vi "CSTK_MCListbox_Designer_Dialog.vi"(10 "MCListbox引用句柄":refnum<vi>, 11 "VI引用输入":refnum<vi>) -> (3 "VI引用输出":refnum<vi>)   [LabVIEW 2015, in "CSTK_MCListbox Designer.lvlib"]
uses:
  CSTK_MCListbox Designer.lvlib
  _CSTK_MCListbox_Designer_ColHdr.ctl
  _CSTK_MCListbox_Designer_ColHdr_Selected.ctl
  _CSTK_MCListbox_Designer_RowAttr.ctl
  <vilib>/Utility/miscctls.llb/LVRowAndColumnTypeDef.ctl
  user32.dll
panel:
  in  "Shutdown":bool
  in  "Minimize":bool
  in  "更新其他属性":bool
  in  "更新表头属性列表":bool
  in  "Refresh":bool
  in  "ArrowDown":bool
  in  "ArrowUp":bool
  in  "Delete":bool
  in  "Create":bool
  in  "行首属性":T1={"宽度"=50, "粗体"=TRUE, "斜体"=FALSE, "对齐"=enum."Center"}
  in  "列":u32
  in  "行":u32
  in  "宽度":u32
  in  "高度":u32
  in  "显示符号":bool
  in  "显示水平线":bool
  in  "显示垂直线":bool
  in  "显示行首":bool
  in  "显示列首":bool
  in  "显示水平滚动条":bool
  in  "显示垂直滚动条":bool
  in  "表头统一属性":T2={"列名称"="", "单元格宽度"=50, "粗体"=TRUE, "斜体"=FALSE, "对齐"=enum."Center"}
  in  "表头属性列表":T3[](array[typedef])
  out "标签名称":string
  # "MCListbox Designer"
  # "列名"
  # "列宽"
  # "粗"
  # "斜"
  # "对齐"
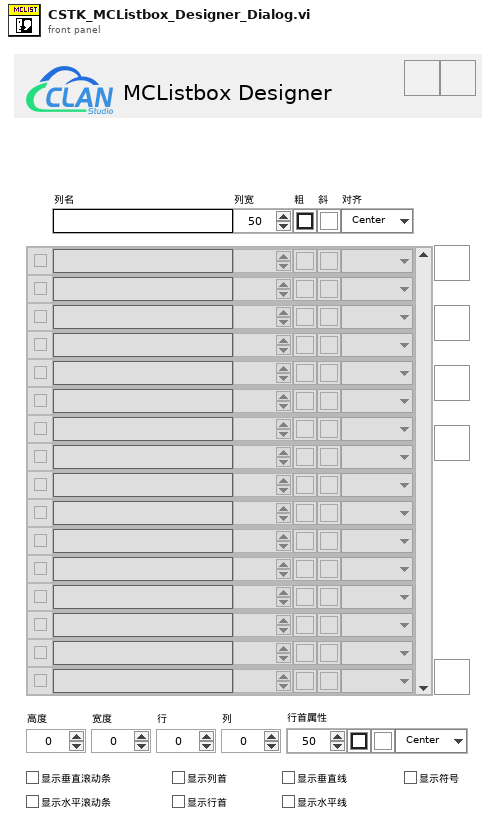
[diagram p1: front panel]
types:
  T1 = typedef "CSTK_MCListbox Designer.lvlib/_CSTK_MCListbox_Designer_RowAttr.ctl" = cluster{"宽度":u32, "粗体":bool, "斜体":bool, "对齐":enum16{"Left", "Center", "Right"}}
  T2 = typedef "CSTK_MCListbox Designer.lvlib/_CSTK_MCListbox_Designer_ColHdr.ctl" = cluster{"列名称":string, "单元格宽度":u32, "粗体":bool, "斜体":bool, "对齐":enum16{"Left", "Center", "Right"}}
  T3 = typedef "CSTK_MCListbox Designer.lvlib/_CSTK_MCListbox_Designer_ColHdr_Selected.ctl" = cluster{"选择":bool, "表头属性":T2}
  T4 = enum32{"Invalid", "Standard", "Closed", "Hidden", "Minimized", "Maximized"}
  T5 = typedef "LVRowAndColumnTypeDef.ctl" = cluster{"Row":i32, "Column":i32}
  T6 = cluster{"高度":refnum<vi>, "宽度":refnum<vi>, "行":refnum<vi>, "列":refnum<vi>, "显示垂直滚动条":refnum<vi>, "显示水平滚动条":refnum<vi>, "显示列首":refnum<vi>, "显示行首":refnum<vi>, "显示垂直线":refnum<vi>, "显示水平线":refnum<vi>, "显示符号":refnum<vi>, "行首属性":refnum<vi>}
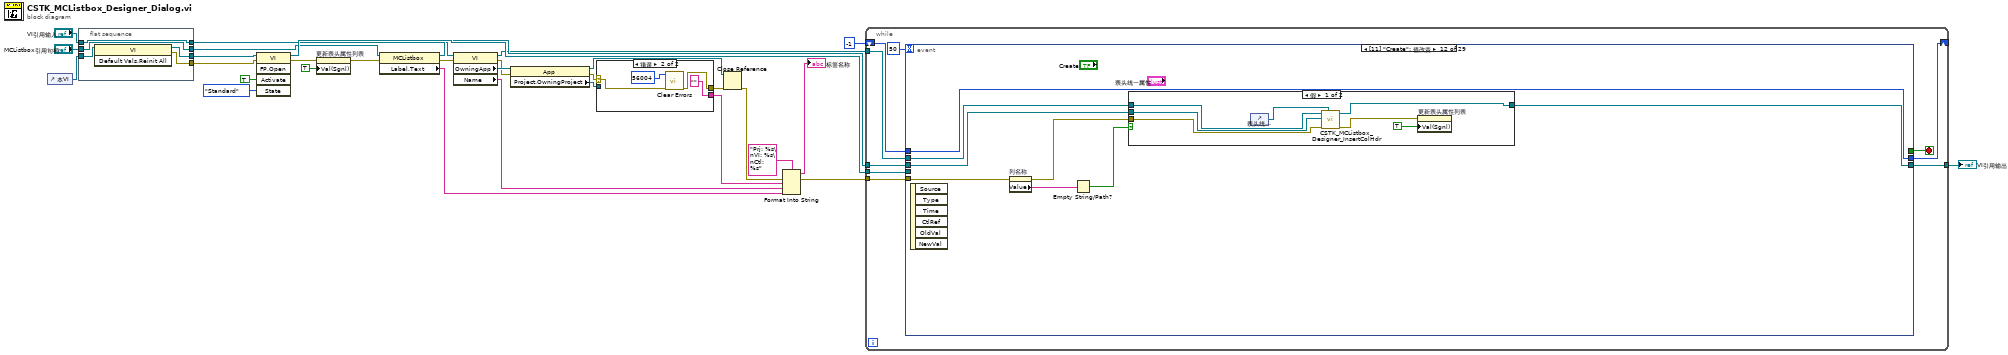
[diagram p0: block diagram]
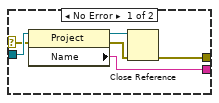
[diagram p2: hidden frame]
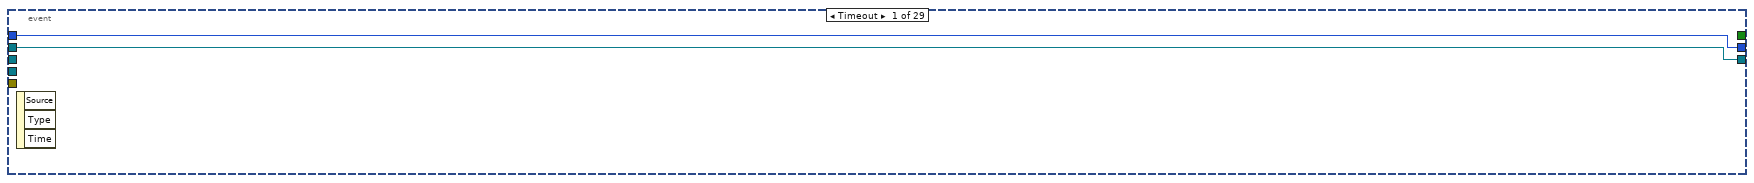
[diagram p3: hidden frame]
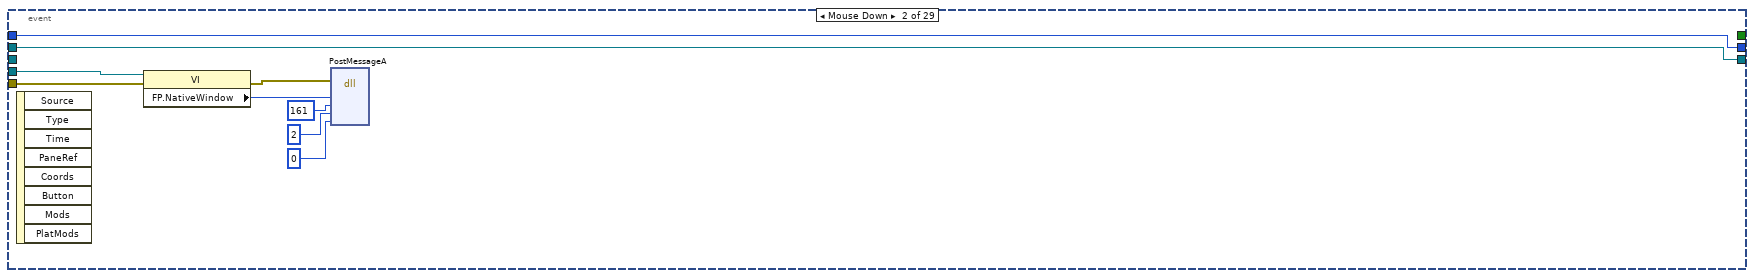
[diagram p4: hidden frame]
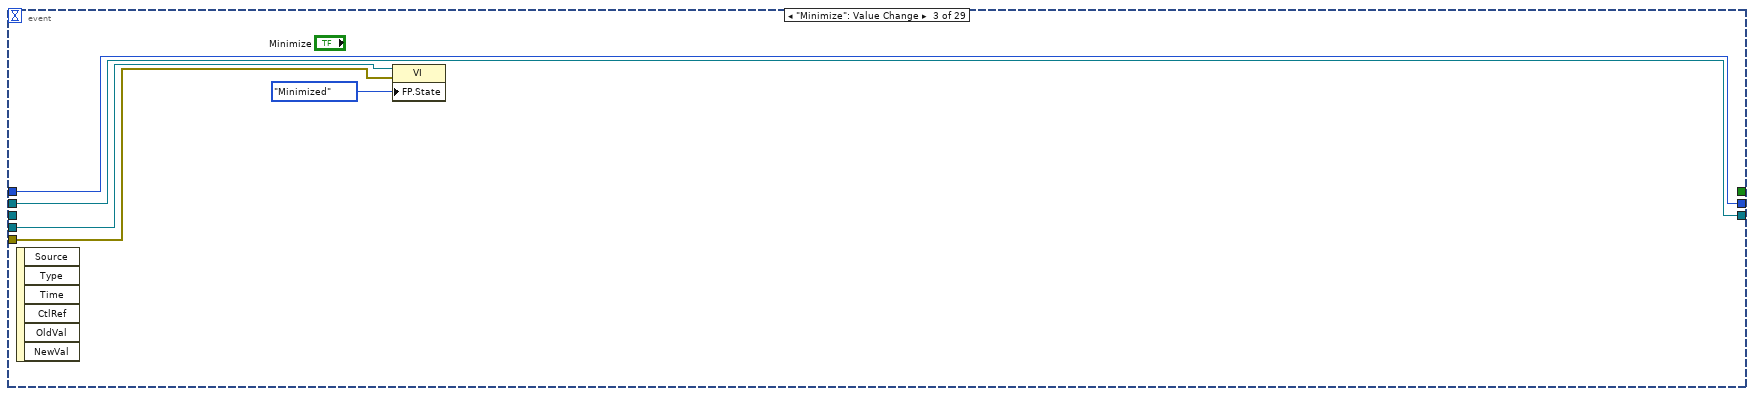
[diagram p5: hidden frame]
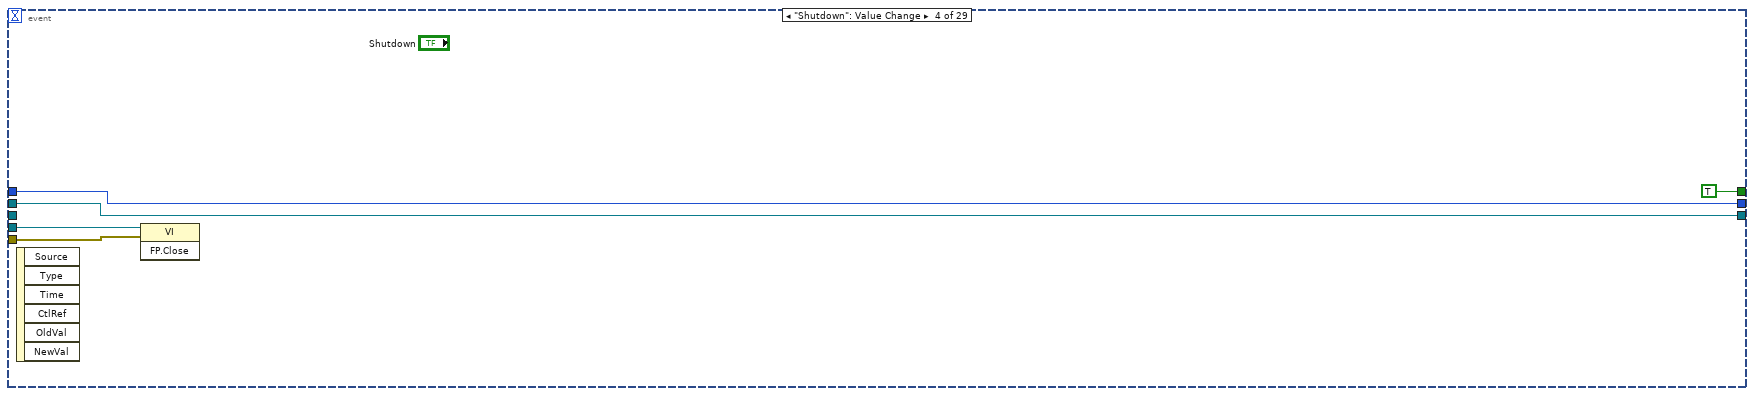
[diagram p6: hidden frame]
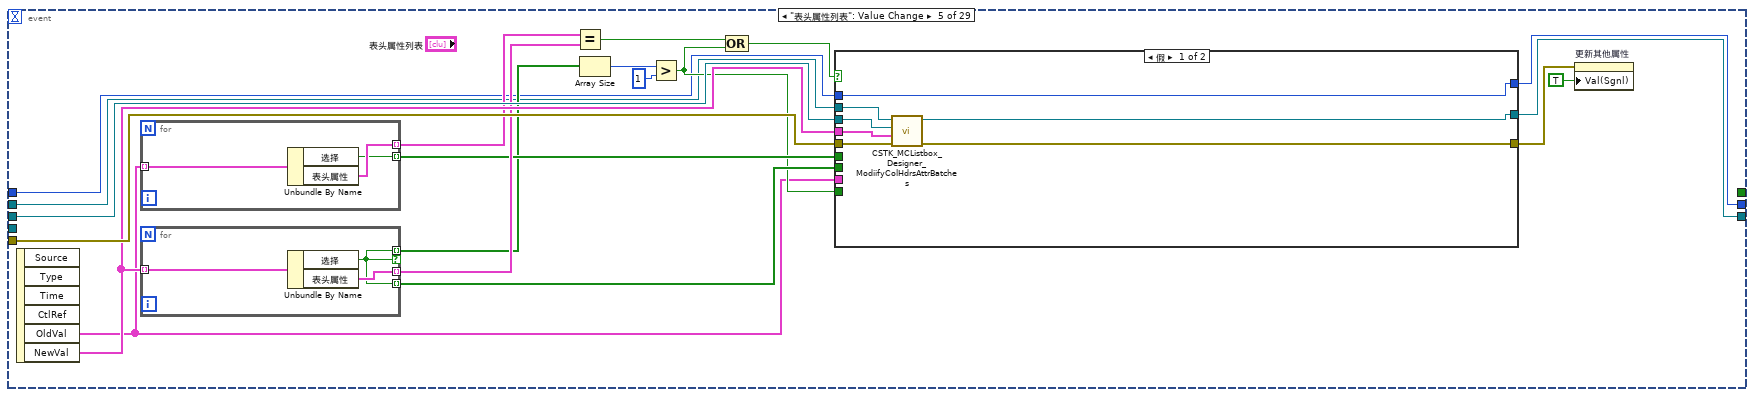
[diagram p7: hidden frame]
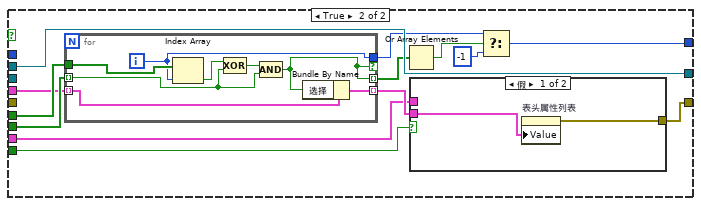
[diagram p8: hidden frame]
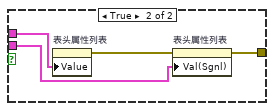
[diagram p9: hidden frame]
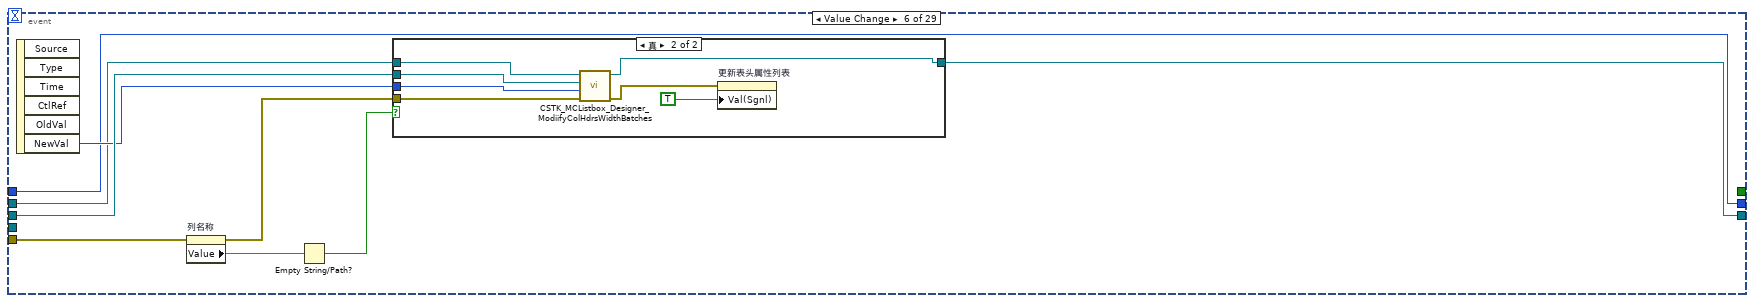
[diagram p10: hidden frame]
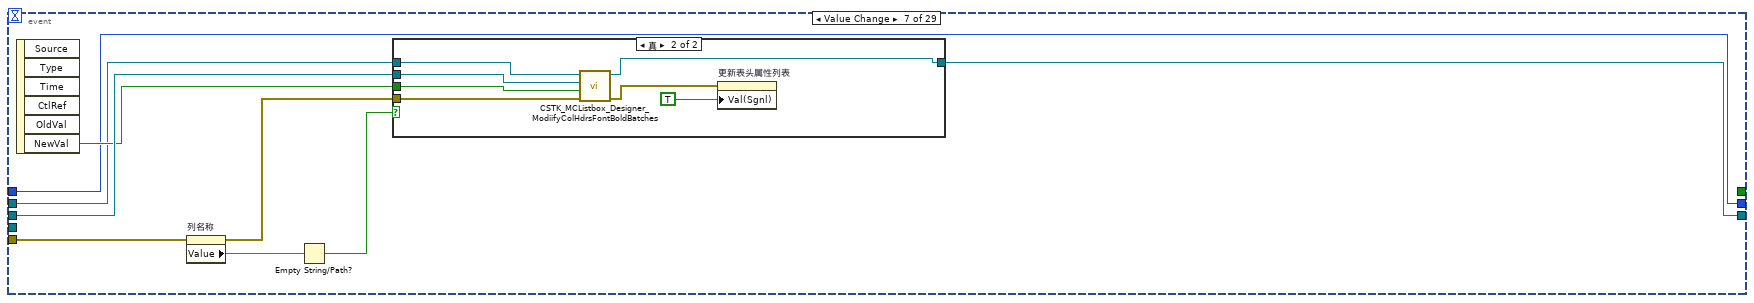
[diagram p12: hidden frame]
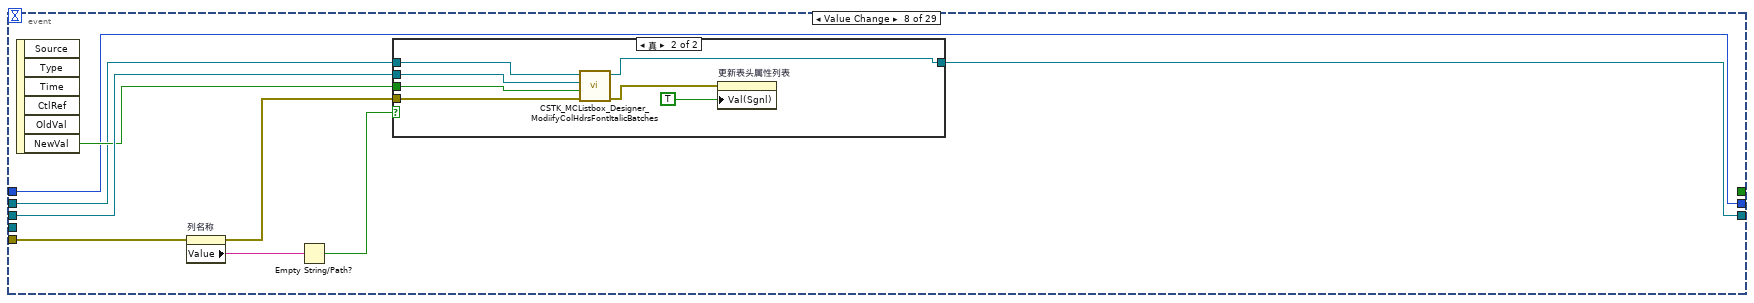
[diagram p14: hidden frame]
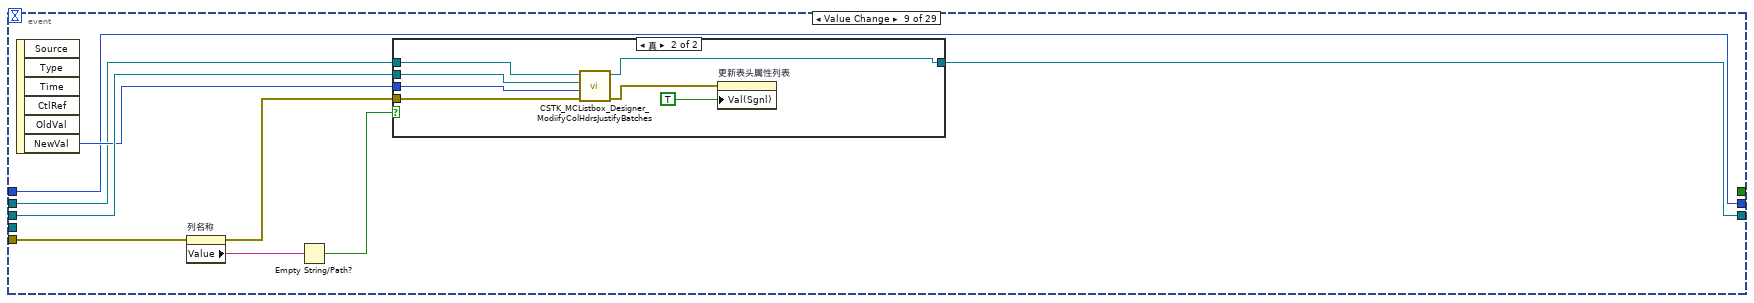
[diagram p16: hidden frame]
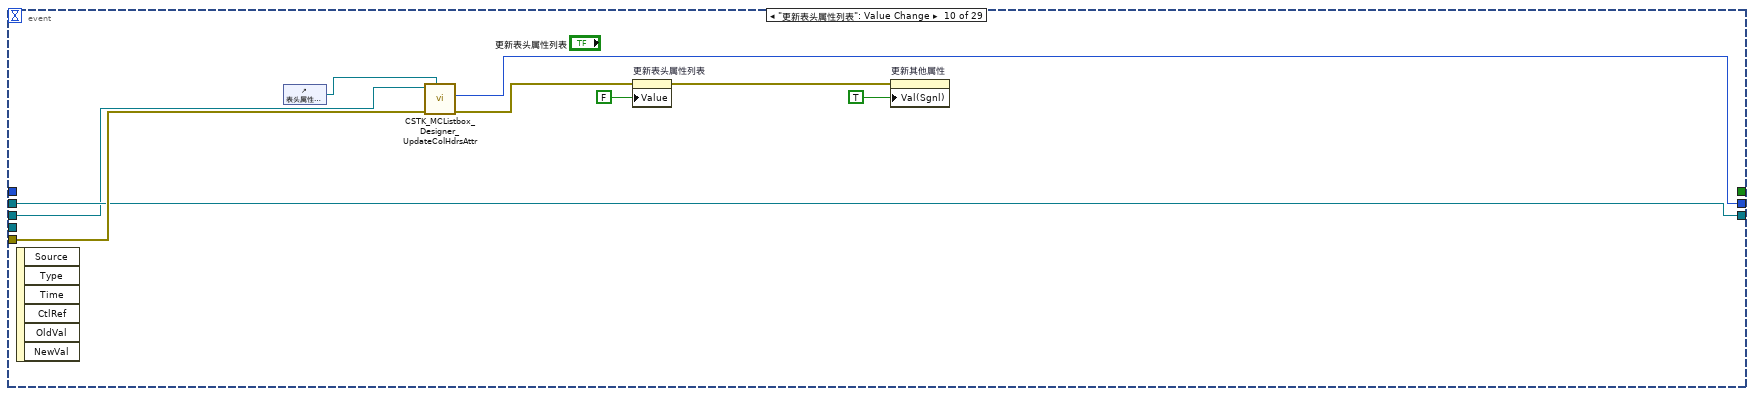
[diagram p18: hidden frame]
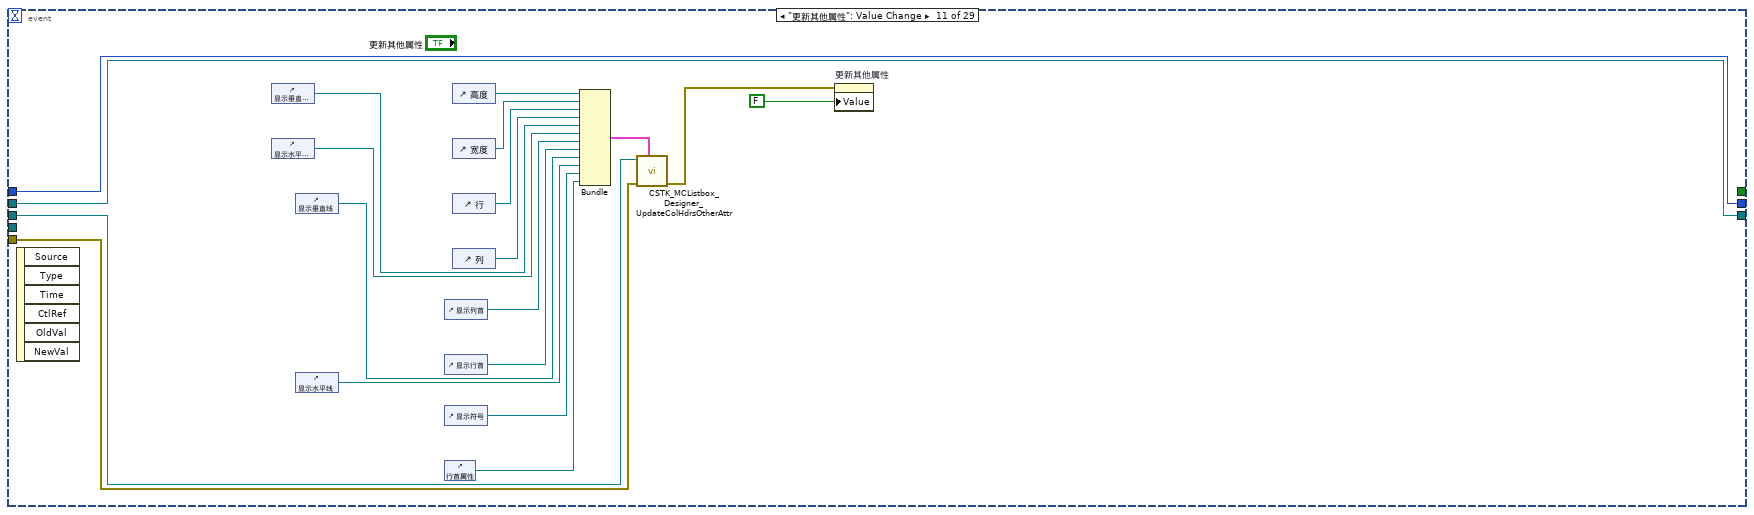
[diagram p19: hidden frame]
diagram:
  n1 = control-ref of="本VI"() -> (w31:refnum<vi>)
  n2 = flat-sequence {
    tunnel: w31 -> [w36]
    tunnel: [w35] -> w30
    tunnel: [w34] -> w29
    tunnel: [w32] -> w19
    tunnel: "MCListbox引用句柄" -> [w32]
    tunnel: [w33] -> w6
    tunnel: "VI引用输入" -> [w33]
    frame #0 {
      n3 = invoke class="VI" method="Default Vals.Reinit All"(reference=w36) -> (reference out=w34:refnum<vi>, error out=w35:errorcluster)  [unwired: 2 in, 1 out]
    }
  }
  n4 = invoke class="VI" method="FP.Open"(reference=w29, error in=w30, "Activate"=TRUE ("激活？"), "State"=T4."Standard" ("状态")) -> (reference out=w20:refnum<vi>, error out=w21:errorcluster)  [unwired: 1 in, 3 out]
  n5 = property on="更新表头属性列表" class="Bool (严格)"(error in=w21, "Val(Sgnl)"=TRUE ("值(信号)")) -> (error out=w1:errorcluster)  [unwired: 1 in, 1 out]
  n6 = property class="MCListbox"(reference=w19, error in=w1) -> (reference out=w18:refnum<vi>, error out=w9:errorcluster, "Label.Text"=w12:string)
  n7 = property class="VI"(reference=w6, error in=w9) -> (reference out=w14:refnum<vi>, error out=w11:errorcluster, "OwningApp"=w17:refnum<vi>, "Name"=w15:string)
  n8 = property class="App"(reference=w17, error in=w11) -> (reference out=w10:refnum<vi>, error out=w4:errorcluster, "Project.OwningProject"=w5:refnum<vi>)
  n9 = case shown="错误" w4 {
    selector: w4 -> [w41 w45]
    tunnel: w5 -> [w42 _]
    tunnel: [w38 "" ("Name")] -> w3
    tunnel: [w37 w44] -> w2
    frame No Error {
      n10 = property class="Project"(reference=w42, error in=w41) -> (reference out=w39:refnum<vi>, error out=w40:errorcluster, "Name"=w38:string)
      n11 = Close Reference(reference=w39, error in (no error)=w40) -> (error out=w37:errorcluster)
    }
    frame Error {
      n12 = call <vilib>:"Clear Errors.vi"("error in (no error)"=w45, "specific error code to clear (0: all)"=56004) -> ("error out"=w44:errorcluster)  [unwired: 4 in, 1 out]
    }
  }
  n13 = Close Reference(reference=w10, error in (no error)=w2) -> (error out=w8:errorcluster)
  n14 = Format Into String(format string="Prj: %s\nVI: %s\nCtl: %s" ("格式字符串"), error in=w8, w3, w15, w12) -> (resulting string=→"标签名称":string, error out=w7:errorcluster)  [unwired: 1 in]
  n15 = while {
    tunnel: w18 -> [w53]
    tunnel: w7 -> [w52]
    tunnel: w14 -> [w50]
    tunnel: [w51] -> w25
    shift-right: [w49] -> _
    shift-left: -1 -> [w48]
    tunnel: w20 -> [w47]
    stop <- w55 stop-if-true
    n16 = event shown="[11] \"Create\": 值改变" {
      selector: _ -> [_ _ _ _ _ _ _ _ _ _ _ _ _ _ _ _ _ _ _ _ _ _ _ _ _ _ _ _ _]
      dyn-events: _ -> [_ _ _ _ _ _ _ _ _ _ _ _ _ _ _ _ _ _ _ _ _ _ _ _ _ _ _ _ _]
      timeout: 50 -> [_ _ _ _ _ _ _ _ _ _ _ _ _ _ _ _ _ _ _ _ _ _ _ _ _ _ _ _ _]
      tunnel: [_ _ _ TRUE _ _ _ _ _ _ _ _ _ _ _ _ _ _ _ _ _ _ _ _ _ _ _ _ TRUE] -> w55
      tunnel: w53 -> [_ _ _ _ w96 w145 w162 w179 w196 w208 w228 w240 w251 w266 w281 _ w302 w309 w316 w323 w330 w337 w344 w351 w358 w365 w372 w383 _]
      tunnel: w52 -> [_ w58 w68 w73 w95 w144 w161 w178 w195 w211 w230 w239 w250 w265 w280 w294 w301 w308 w315 w322 w329 w336 w343 w350 w357 w364 w371 w382 _]
      tunnel: [w57 w66 w71 w76 w79 w138 w155 w172 w189 w210 w229 w235 w252 w267 w282 w297 w304 w311 w318 w325 w332 w339 w346 w353 w360 w367 w374 w386 w388] -> w51
      tunnel: w50 -> [w57 w66 w71 w76 w80 w139 w156 w173 w190 w210 w229 w236 w253 w268 w283 w297 w304 w311 w318 w325 w332 w339 w346 w353 w360 w367 w374 w386 w388]
      tunnel: [w56 w65 w70 w75 w81 w137 w154 w171 w188 w209 w227 w233 w249 w264 w279 w296 w303 w310 w317 w324 w331 w338 w345 w352 w359 w366 w373 w385 w387] -> w49
      tunnel: w48 -> [w56 w65 w70 w75 w82 w137 w154 w171 w188 _ w227 w233 w249 w264 w279 w296 w303 w310 w317 w324 w331 w338 w345 w352 w359 w366 w373 w385 w387]
      tunnel: w47 -> [_ w59 w67 w74 _ _ _ _ _ _ _ _ _ _ _ _ _ _ _ _ _ _ _ _ _ _ _ _ _]
      event Timeout {
        n17 = event-data() -> ()  [unwired: 1 in, 3 out]
      }
      event Mouse Down {
        n18 = event-data() -> ()  [unwired: 1 in, 8 out]
        n19 = property class="VI"(reference=w59, error in=w58) -> (error out=w60:errorcluster, "FP.NativeWindow"=w61:u64)  [unwired: 1 out]
        n20 = dll-call lib="user32.dll" fn="PostMessageA"(error in=w60, "hWnd"=w61, "Msg"=161, "wParam"=2, "IParam"=0 ("wParam")) -> ()  [unwired: 7 in, 2 out]
      }
      event "Minimize": Value Change {
        n21 = event-data() -> ()  [unwired: 1 in, 6 out]
        n22 = property class="VI"(reference=w67, error in=w68, "FP.State"=T4."Minimized" ("Front Panel Window:State")) -> ()  [unwired: 2 out]
      }
      event "Shutdown": Value Change {
        n23 = event-data() -> ()  [unwired: 1 in, 6 out]
        n24 = invoke class="VI" method="FP.Close"(reference=w74, error in=w73) -> ()  [unwired: 1 in, 3 out]
      }
      event "表头属性列表": Value Change {
        n25 = event-data() -> ("OldVal"=w83:T3[], "NewVal"=w94:T3[])  [unwired: 1 in, 4 out]
        n26 = for {
          tunnel: w83 -> [w102] mode=indexing
          tunnel: [w101] -> w93 mode=indexing
          tunnel: [w100] -> w90 mode=indexing
          n27 = Unbundle By Name(w102) -> ("选择"=w100:bool, "表头属性"=w101:T2)
        }
        n28 = for {
          tunnel: w94 -> [w99] mode=indexing
          tunnel: [w98] -> w92 mode=indexing
          tunnel: [w97] -> w89 mode=indexing
          tunnel: [w97] -> w88 mode=indexing if=w97
          n29 = Unbundle By Name(w99) -> ("选择"=w97:bool, "表头属性"=w98:T2)
        }
        n30 = Equal?(x=w93, y=w92) -> (x = y?=w91:bool)
        n31 = Array Size(array=w88) -> (size(s)=w86:i32)
        n32 = Greater?(x=w86, y=1) -> (0:w84:bool)
        n33 = Compound Arithmetic op=OR ("复合运算")(w91, w84) -> (w87:bool)
        n34 = case shown="假" w87 {
          tunnel: w96 -> [w104 _]
          tunnel: w94 -> [w109 w120]
          tunnel: w80 -> [w105 w116]
          tunnel: w95 -> [w108 _]
          tunnel: w90 -> [_ w122]
          tunnel: w89 -> [_ w121]
          tunnel: w84 -> [_ w118]
          tunnel: w83 -> [_ w117]
          tunnel: w82 -> [w107 _]
          tunnel: [w107 w112] -> w81
          tunnel: [w106 w116] -> w79
          tunnel: [w103 w110] -> w77
          frame False {
            n35 = call "CSTK_MCListbox_Designer_ModiifyColHdrsAttrBatches.vi"("错误输入（无错误）"=w108, "Attr"=w109, "MulticolumnListbox输入"=w104, "VI输入"=w105) -> ("错误输出"=w103:errorcluster, "VI输出"=w106:refnum<vi>)  [unwired: 6 in]
          }
          frame True {
            n36 = for {
              tunnel: w122 -> [w135]
              tunnel: w121 -> [w134] mode=indexing
              tunnel: w120 -> [w132] mode=indexing
              tunnel: [w131] -> w119 mode=indexing
              tunnel: [w130] -> w113 if=w129
              tunnel: [w129] -> w115 mode=indexing
              i -> [w130]
              n37 = Index Array(array=w135, index=w130) -> (element=w133:bool)
              n38 = Compound Arithmetic op=XOR ("复合运算")(w133, w134) -> (w136:bool)
              n39 = Compound Arithmetic op=AND ("复合运算")(w136, w134) -> (w129:bool)
              n40 = Bundle By Name(cluster=w132, "选择"=w129) -> (w131:T3)
            }
            n41 = Or Array Elements(Boolean array=w115) -> (logical OR=w114:bool)
            n42 = case shown="假" w118 {
              tunnel: w119 -> [w124 w127]
              tunnel: w117 -> [_ w126]
              tunnel: [w123 w125] -> w110
              frame False {
                n43 = property on="表头属性列表" class="Arr (严格)"("Value"=w124) -> (error out=w123:errorcluster)  [unwired: 2 in, 1 out]
              }
              frame True {
                n44 = property on="表头属性列表" class="Arr (严格)"("Value"=w126) -> (error out=w128:errorcluster)  [unwired: 2 in, 1 out]
                n45 = property on="表头属性列表" class="Arr (严格)"(error in=w128, "Val(Sgnl)"=w127) -> (error out=w125:errorcluster)  [unwired: 1 in, 1 out]
              }
            }
            n46 = Select(t=w113, s=w114, f=-1) -> (s? t:f=w112:i32)
          }
        }
        n47 = property on="更新其他属性" class="Bool (严格)"(error in=w77, "Val(Sgnl)"=TRUE ("值(信号)")) -> ()  [unwired: 1 in, 2 out]
      }
      event Value Change {
        n48 = event-data() -> ("NewVal"=w140:u32)  [unwired: 1 in, 5 out]
        n49 = property on="列名称" class="Str"(error in=w144) -> (error out=w143:errorcluster, "Value"=w142:string)  [unwired: 1 in, 1 out]
        n50 = Empty String/Path?(string/path=w142) -> (empty?=w141:bool)
        n51 = case shown="真" w141 {
          tunnel: w145 -> [_ w147]
          tunnel: w143 -> [_ w152]
          tunnel: w140 -> [_ w153]
          tunnel: w139 -> [w146 w148]
          tunnel: [w146 w151] -> w138
          frame False {
          }
          frame True {
            n52 = call "CSTK_MCListbox_Designer_ModiifyColHdrsWidthBatches.vi"("错误输入（无错误）"=w152, "Width"=w153, "MulticolumnListbox输入"=w147, "VI输入"=w148) -> ("错误输出"=w149:errorcluster, "VI输出"=w151:refnum<vi>)  [unwired: 6 in]
            n53 = property on="更新表头属性列表" class="Bool (严格)"(error in=w149, "Val(Sgnl)"=TRUE ("值(信号)")) -> ()  [unwired: 1 in, 2 out]
          }
        }
      }
      event Value Change {
        n54 = event-data() -> ("NewVal"=w157:bool)  [unwired: 1 in, 5 out]
        n55 = property on="列名称" class="Str"(error in=w161) -> (error out=w160:errorcluster, "Value"=w159:string)  [unwired: 1 in, 1 out]
        n56 = Empty String/Path?(string/path=w159) -> (empty?=w158:bool)
        n57 = case shown="真" w158 {
          tunnel: w162 -> [_ w164]
          tunnel: w160 -> [_ w169]
          tunnel: w157 -> [_ w170]
          tunnel: w156 -> [w163 w165]
          tunnel: [w163 w168] -> w155
          frame False {
          }
          frame True {
            n58 = call "CSTK_MCListbox_Designer_ModiifyColHdrsFontBoldBatches.vi"("错误输入（无错误）"=w169, "FontBold"=w170, "MulticolumnListbox输入"=w164, "VI输入"=w165) -> ("错误输出"=w166:errorcluster, "VI输出"=w168:refnum<vi>)  [unwired: 6 in]
            n59 = property on="更新表头属性列表" class="Bool (严格)"(error in=w166, "Val(Sgnl)"=TRUE ("值(信号)")) -> ()  [unwired: 1 in, 2 out]
          }
        }
      }
      event Value Change {
        n60 = event-data() -> ("NewVal"=w174:bool)  [unwired: 1 in, 5 out]
        n61 = property on="列名称" class="Str"(error in=w178) -> (error out=w177:errorcluster, "Value"=w176:string)  [unwired: 1 in, 1 out]
        n62 = Empty String/Path?(string/path=w176) -> (empty?=w175:bool)
        n63 = case shown="真" w175 {
          tunnel: w179 -> [_ w181]
          tunnel: w177 -> [_ w186]
          tunnel: w174 -> [_ w187]
          tunnel: w173 -> [w180 w182]
          tunnel: [w180 w185] -> w172
          frame False {
          }
          frame True {
            n64 = call "CSTK_MCListbox_Designer_ModiifyColHdrsFontItalicBatches.vi"("错误输入（无错误）"=w186, "FontItalic"=w187, "MulticolumnListbox输入"=w181, "VI输入"=w182) -> ("错误输出"=w183:errorcluster, "VI输出"=w185:refnum<vi>)  [unwired: 6 in]
            n65 = property on="更新表头属性列表" class="Bool (严格)"(error in=w183, "Val(Sgnl)"=TRUE ("值(信号)")) -> ()  [unwired: 1 in, 2 out]
          }
        }
      }
      event Value Change {
        n66 = event-data() -> ("NewVal"=w191:enum16{"Left", "Center", "Right"})  [unwired: 1 in, 5 out]
        n67 = property on="列名称" class="Str"(error in=w195) -> (error out=w194:errorcluster, "Value"=w193:string)  [unwired: 1 in, 1 out]
        n68 = Empty String/Path?(string/path=w193) -> (empty?=w192:bool)
        n69 = case shown="真" w192 {
          tunnel: w196 -> [_ w199]
          tunnel: w194 -> [_ w203]
          tunnel: w191 -> [_ w204]
          tunnel: w190 -> [w197 w198]
          tunnel: [w197 w202] -> w189
          frame False {
          }
          frame True {
            n70 = call "CSTK_MCListbox_Designer_ModiifyColHdrsJustifyBatches.vi"("错误输入（无错误）"=w203, "Justify"=w204, "MulticolumnListbox输入"=w199, "VI输入"=w198) -> ("错误输出"=w200:errorcluster, "VI输出"=w202:refnum<vi>)  [unwired: 6 in]
            n71 = property on="更新表头属性列表" class="Bool (严格)"(error in=w200, "Val(Sgnl)"=TRUE ("值(信号)")) -> ()  [unwired: 1 in, 2 out]
          }
        }
      }
      event "更新表头属性列表": Value Change {
        n72 = event-data() -> ()  [unwired: 1 in, 6 out]
        n73 = control-ref of="表头属性列表"() -> (w205:refnum<vi>)
        n74 = call "CSTK_MCListbox_Designer_UpdateColHdrsAttr.vi"("表头属性列表输入"=w205, "错误输入（无错误）"=w211, "MCListbox引用句柄"=w208) -> ("错误输出"=w213:errorcluster, "Selected Index"=w209:i32)  [unwired: 7 in]
        n75 = property on="更新表头属性列表" class="Bool (严格)"(error in=w213, "Value"=FALSE ("更新表头属性列表")) -> (error out=w207:errorcluster)  [unwired: 1 in, 1 out]
        n76 = property on="更新其他属性" class="Bool (严格)"(error in=w207, "Val(Sgnl)"=TRUE ("值(信号)")) -> ()  [unwired: 1 in, 2 out]
      }
      event "更新其他属性": Value Change {
        n77 = event-data() -> ()  [unwired: 1 in, 6 out]
        n78 = control-ref of="显示垂直滚动条"() -> (w220:refnum<vi>)
        n79 = control-ref of="显示水平滚动条"() -> (w221:refnum<vi>)
        n80 = control-ref of="显示垂直线"() -> (w224:refnum<vi>)
        n81 = control-ref of="显示水平线"() -> (w225:refnum<vi>)
        n82 = control-ref of="显示列首"() -> (w222:refnum<vi>)
        n83 = control-ref of="显示行首"() -> (w223:refnum<vi>)
        n84 = control-ref of="显示符号"() -> (w226:refnum<vi>)
        n85 = control-ref of="行首属性"() -> (w214:refnum<vi>)
        n86 = control-ref of="高度"() -> (w216:refnum<vi>)
        n87 = control-ref of="宽度"() -> (w217:refnum<vi>)
        n88 = control-ref of="行"() -> (w218:refnum<vi>)
        n89 = control-ref of="列"() -> (w219:refnum<vi>)
        n90 = Bundle("高度"=w216, "宽度"=w217, "行"=w218, "列"=w219, "显示垂直滚动条"=w220, "显示水平滚动条"=w221, "显示列首"=w222, "显示行首"=w223, "显示垂直线"=w224, "显示水平线"=w225, "显示符号"=w226, "行首属性"=w214) -> (w215:T6)  [unwired: 1 in]
        n91 = call "CSTK_MCListbox_Designer_UpdateColHdrsOtherAttr.vi"("引用输入"=w215, "错误输入（无错误）"=w230, "MCListbox引用句柄"=w228) -> ("错误输出"=w232:errorcluster)  [unwired: 8 in]
        n92 = property on="更新其他属性" class="Bool (严格)"(error in=w232, "Value"=FALSE ("更新表头属性列表")) -> ()  [unwired: 1 in, 2 out]
      }
      event "Create": Value Change {
        n93 = event-data() -> ()  [unwired: 1 in, 6 out]
        n94 = property on="列名称" class="Str"(error in=w239) -> (error out=w238:errorcluster, "Value"=w234:string)  [unwired: 1 in, 1 out]
        n95 = Empty String/Path?(string/path=w234) -> (empty?=w237:bool)
        n96 = case shown="假" w237 {
          tunnel: w240 -> [w245 _]
          tunnel: w238 -> [w247 _]
          tunnel: w236 -> [w242 w248]
          tunnel: [w246 w248] -> w235
          frame False {
            n97 = control-ref of="表头统一属性"() -> (w241:refnum<vi>)
            n98 = call "CSTK_MCListbox_Designer_InsertColHdr.vi"("表头统一属性输入"=w241, "错误输入（无错误）"=w247, "MCListbox引用句柄"=w245, "VI输入"=w242) -> ("错误输出"=w243:errorcluster, "VI输出"=w246:refnum<vi>)  [unwired: 6 in]
            n99 = property on="更新表头属性列表" class="Bool (严格)"(error in=w243, "Val(Sgnl)"=TRUE ("值(信号)")) -> ()  [unwired: 1 in, 2 out]
          }
          frame True {
          }
        }
      }
      event "Delete": Value Change {
        n100 = event-data() -> ()  [unwired: 1 in, 6 out]
        n101 = Greater Or Equal To 0?(x=w249) -> (x >= 0?=w254:bool)
        n102 = case shown="真" w254 {
          tunnel: w251 -> [_ w259]
          tunnel: w250 -> [_ w263]
          tunnel: w253 -> [w255 w257]
          tunnel: [w255 w262] -> w252
          tunnel: w249 -> [_ w256]
          frame False {
          }
          frame True {
            n103 = control-ref of="表头属性列表"() -> (w258:refnum<vi>)
            n104 = call "CSTK_MCListbox_Designer_DeleteColHdr.vi"("表头属性列表输入"=w258, "错误输入（无错误）"=w263, "Selected Index"=w256, "MCListbox引用句柄"=w259, "VI输入"=w257) -> ("错误输出"=w260:errorcluster, "VI输出"=w262:refnum<vi>)  [unwired: 5 in]
            n105 = property on="更新表头属性列表" class="Bool (严格)"(error in=w260, "Val(Sgnl)"=TRUE ("值(信号)")) -> ()  [unwired: 1 in, 2 out]
          }
        }
      }
      event "ArrowUp": Value Change {
        n106 = event-data() -> ()  [unwired: 1 in, 6 out]
        n107 = Greater Or Equal To 0?(x=w264) -> (x >= 0?=w269:bool)
        n108 = case shown="真" w269 {
          tunnel: w266 -> [_ w274]
          tunnel: w265 -> [_ w278]
          tunnel: w268 -> [w270 w272]
          tunnel: [w270 w277] -> w267
          tunnel: w264 -> [_ w271]
          frame False {
          }
          frame True {
            n109 = control-ref of="表头属性列表"() -> (w273:refnum<vi>)
            n110 = call "CSTK_MCListbox_Designer_MoveUpColHdr.vi"("表头属性列表输入"=w273, "错误输入（无错误）"=w278, "Selected Index"=w271, "MCListbox引用句柄"=w274, "VI输入"=w272) -> ("错误输出"=w275:errorcluster, "VI输出"=w277:refnum<vi>)  [unwired: 5 in]
            n111 = property on="更新表头属性列表" class="Bool (严格)"(error in=w275, "Val(Sgnl)"=TRUE ("值(信号)")) -> ()  [unwired: 1 in, 2 out]
          }
        }
      }
      event "ArrowDown": Value Change {
        n112 = event-data() -> ()  [unwired: 1 in, 6 out]
        n113 = Greater Or Equal To 0?(x=w279) -> (x >= 0?=w284:bool)
        n114 = case shown="真" w284 {
          tunnel: w281 -> [_ w289]
          tunnel: w280 -> [_ w293]
          tunnel: w283 -> [w285 w287]
          tunnel: [w285 w292] -> w282
          tunnel: w279 -> [_ w286]
          frame False {
          }
          frame True {
            n115 = control-ref of="表头属性列表"() -> (w288:refnum<vi>)
            n116 = call "CSTK_MCListbox_Designer_MoveDownColHdr.vi"("表头属性列表输入"=w288, "错误输入（无错误）"=w293, "Selected Index"=w286, "MCListbox引用句柄"=w289, "VI输入"=w287) -> ("错误输出"=w290:errorcluster, "VI输出"=w292:refnum<vi>)  [unwired: 5 in]
            n117 = property on="更新表头属性列表" class="Bool (严格)"(error in=w290, "Val(Sgnl)"=TRUE ("值(信号)")) -> ()  [unwired: 1 in, 2 out]
          }
        }
      }
      event "Refresh": Value Change {
        n118 = event-data() -> ()  [unwired: 1 in, 6 out]
        n119 = property on="更新表头属性列表" class="Bool (严格)"(error in=w294, "Val(Sgnl)"=TRUE ("值(信号)")) -> ()  [unwired: 1 in, 2 out]
      }
      event "高度": Value Change {
        n120 = event-data() -> ("NewVal"=w300:u32)  [unwired: 1 in, 5 out]
        n121 = property class="MCListbox"(reference=w302, error in=w301, "Height"=w300) -> (error out=w298:errorcluster)  [unwired: 1 out]
        n122 = property on="更新其他属性" class="Bool (严格)"(error in=w298, "Val(Sgnl)"=TRUE ("值(信号)")) -> ()  [unwired: 1 in, 2 out]
      }
      event "宽度": Value Change {
        n123 = event-data() -> ("NewVal"=w307:u32)  [unwired: 1 in, 5 out]
        n124 = property class="MCListbox"(reference=w309, error in=w308, "Width"=w307) -> (error out=w305:errorcluster)  [unwired: 1 out]
        n125 = property on="更新其他属性" class="Bool (严格)"(error in=w305, "Val(Sgnl)"=TRUE ("值(信号)")) -> ()  [unwired: 1 in, 2 out]
      }
      event "行": Value Change {
        n126 = event-data() -> ("NewVal"=w314:u32)  [unwired: 1 in, 5 out]
        n127 = property class="MCListbox"(reference=w316, error in=w315, "NumRows"=w314) -> (error out=w312:errorcluster)  [unwired: 1 out]
        n128 = property on="更新其他属性" class="Bool (严格)"(error in=w312, "Val(Sgnl)"=TRUE ("值(信号)")) -> ()  [unwired: 1 in, 2 out]
      }
      event "列": Value Change {
        n129 = event-data() -> ("NewVal"=w321:u32)  [unwired: 1 in, 5 out]
        n130 = property class="MCListbox"(reference=w323, error in=w322, "NumCols"=w321) -> (error out=w319:errorcluster)  [unwired: 1 out]
        n131 = property on="更新其他属性" class="Bool (严格)"(error in=w319, "Val(Sgnl)"=TRUE ("值(信号)")) -> ()  [unwired: 1 in, 2 out]
      }
      event "显示垂直滚动条": Value Change {
        n132 = event-data() -> ("NewVal"=w328:bool)  [unwired: 1 in, 5 out]
        n133 = property class="MCListbox"(reference=w330, error in=w329, "VScrollVis"=w328) -> (error out=w326:errorcluster)  [unwired: 1 out]
        n134 = property on="更新其他属性" class="Bool (严格)"(error in=w326, "Val(Sgnl)"=TRUE ("值(信号)")) -> ()  [unwired: 1 in, 2 out]
      }
      event "显示水平滚动条": Value Change {
        n135 = event-data() -> ("NewVal"=w335:bool)  [unwired: 1 in, 5 out]
        n136 = property class="MCListbox"(reference=w337, error in=w336, "HScrollVis"=w335) -> (error out=w333:errorcluster)  [unwired: 1 out]
        n137 = property on="更新其他属性" class="Bool (严格)"(error in=w333, "Val(Sgnl)"=TRUE ("值(信号)")) -> ()  [unwired: 1 in, 2 out]
      }
      event "显示列首": Value Change {
        n138 = event-data() -> ("NewVal"=w342:bool)  [unwired: 1 in, 5 out]
        n139 = property class="MCListbox"(reference=w344, error in=w343, "ColHdrVis"=w342) -> (error out=w340:errorcluster)  [unwired: 1 out]
        n140 = property on="更新其他属性" class="Bool (严格)"(error in=w340, "Val(Sgnl)"=TRUE ("值(信号)")) -> ()  [unwired: 1 in, 2 out]
      }
      event "显示行首": Value Change {
        n141 = event-data() -> ("NewVal"=w349:bool)  [unwired: 1 in, 5 out]
        n142 = property class="MCListbox"(reference=w351, error in=w350, "RowHdrVis"=w349) -> (error out=w347:errorcluster)  [unwired: 1 out]
        n143 = property on="更新其他属性" class="Bool (严格)"(error in=w347, "Val(Sgnl)"=TRUE ("值(信号)")) -> ()  [unwired: 1 in, 2 out]
      }
      event "显示垂直线": Value Change {
        n144 = event-data() -> ("NewVal"=w356:bool)  [unwired: 1 in, 5 out]
        n145 = property class="MCListbox"(reference=w358, error in=w357, "Vertical Lines Visible"=w356) -> (error out=w354:errorcluster)  [unwired: 1 out]
        n146 = property on="更新其他属性" class="Bool (严格)"(error in=w354, "Val(Sgnl)"=TRUE ("值(信号)")) -> ()  [unwired: 1 in, 2 out]
      }
      event "显示水平线": Value Change {
        n147 = event-data() -> ("NewVal"=w363:bool)  [unwired: 1 in, 5 out]
        n148 = property class="MCListbox"(reference=w365, error in=w364, "Horizontal Lines Visible"=w363) -> (error out=w361:errorcluster)  [unwired: 1 out]
        n149 = property on="更新其他属性" class="Bool (严格)"(error in=w361, "Val(Sgnl)"=TRUE ("值(信号)")) -> ()  [unwired: 1 in, 2 out]
      }
      event "显示符号": Value Change {
        n150 = event-data() -> ("NewVal"=w370:bool)  [unwired: 1 in, 5 out]
        n151 = property class="MCListbox"(reference=w372, error in=w371, "Symbols Vis"=w370) -> (error out=w368:errorcluster)  [unwired: 1 out]
        n152 = property on="更新其他属性" class="Bool (严格)"(error in=w368, "Val(Sgnl)"=TRUE ("值(信号)")) -> ()  [unwired: 1 in, 2 out]
      }
      event Value Change {
        n153 = event-data() -> ("NewVal"=w379:T1)  [unwired: 1 in, 5 out]
        n154 = Unbundle By Name(w379) -> ("宽度"=w378:u32, "粗体"=w377:bool, "斜体"=w375:bool, "对齐"=w376:enum16{"Left", "Center", "Right"})
        n155 = property class="MCListbox"(reference=w383, error in=w382, "ActiveCell"=T5 {"Row"=-2, "Column"=-1} ("活动单元格:活动单元格"), "Width"=w378, "CellFontBold"=w377, "CellFontItalic"=w375, "Justify"=w376) -> (error out=w381:errorcluster)  [unwired: 1 out]
        n156 = property on="更新其他属性" class="Bool (严格)"(error in=w381, "Val(Sgnl)"=TRUE ("值(信号)")) -> ()  [unwired: 1 in, 2 out]
      }
      event Panel Close {
        n157 = event-data() -> ()  [unwired: 1 in, 4 out]
      }
    }
  }
  "VI引用输出" <- w25
